vi "AuMT8852B Tester Firmware and Date stamp.vi"(8 "error in (no error)":errorcluster, 11 "VISA session":refnum<visa-resource-name>) -> (0 "error out":errorcluster, 2 "error code":i32, 3 "VISA session out":refnum<visa-resource-name>, 4 "Tester Firmware Date Stamp":T1)   [LabVIEW 2017]
doc: "Anritsu MT8852B Bluetooth Tester\n\nObtains the version and date stamp information for all the modules with the Anritsu Bluetooth test set.\n\nTester Information:\nBase Band boot code date and time stamp.\nBase Band ARM code date and time stamp.\nBase Band FPGA date and time stamp.\nRF FPGA date and time stamp.\nDSP software version number."
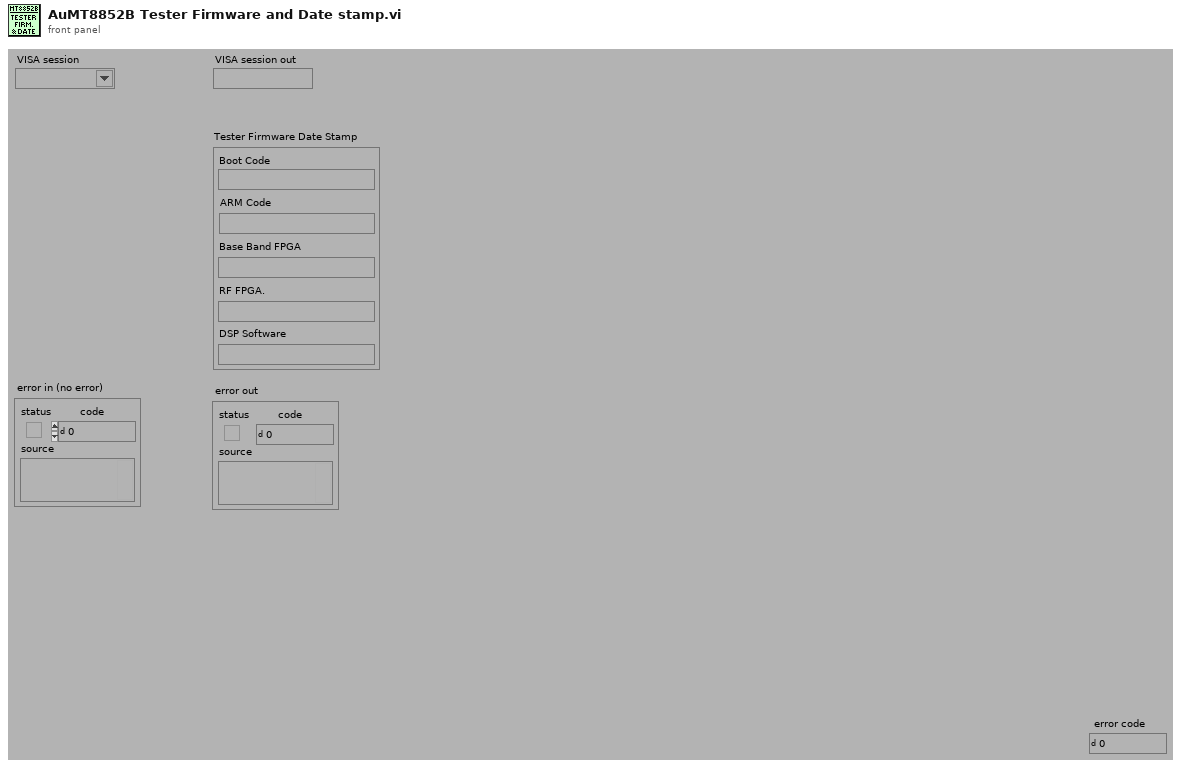
[diagram p1: front panel]
types:
  T1 = cluster{"ARM Code":string, "Base Band FPGA":string, "DSP Software":string, "RF FPGA.":string, "Boot Code":string}
  T2 = enum16{"Simulate", "Range check", "Cache", "Query instrument status"}
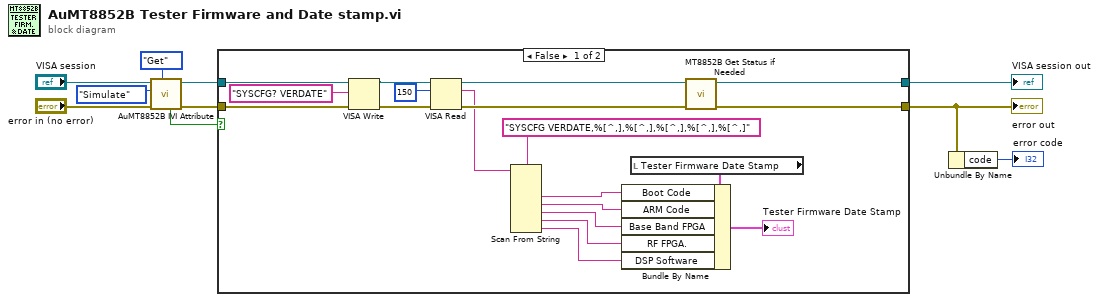
[diagram p0: block diagram]
diagram:
  n1 = call <instrlib>:"AuMT8852B IVI Attribute.vi"("Set/Get (Set)"=enum16{"Set", "Get"}."Get", "error in (no error)"="error in (no error)", "Flag (Simulate)"=T2."Simulate", "VISA session"="VISA session") -> ("error out"=w7:errorcluster, "VISA session out"=w9:refnum<visa-resource-name>, "Value out"=w3:bool)  [unwired: 5 in]
  n2 = case shown="False" w3 {
    tunnel: [w21 w31] -> w10
    tunnel: [w20 w30] -> w1
    tunnel: w9 -> [w28 w31]
    tunnel: w7 -> [w27 w30]
    frame False {
      n3 = VISA Write(VISA resource name=w28, write buffer="SYSCFG? VERDATE" ("write buffer (\"\")"), error in (no error)=w27) -> (VISA resource name out=w26:refnum<visa-resource-name>, error out=w25:errorcluster)  [unwired: 1 out]
      n4 = VISA Read(VISA resource name=w26, byte count=u32 150 ("byte count (0)"), error in (no error)=w25) -> (VISA resource name out=w18:refnum<visa-resource-name>, read buffer=w16:string, error out=w19:errorcluster)  [unwired: 1 out]
      n5 = Scan From String(format string="SYSCFG VERDATE,%[^,],%[^,],%[^,],%[^,],%[^,]" ("write buffer (\"\")"), input string=w16) -> (output 1=w15:string, output 2=w12:string, output 3=w14:string, output 4=w13:string, output 5=w11:string)  [unwired: 7 in, 3 out]
      n6 = local read "Tester Firmware Date Stamp"() -> (w23:T1)
      n7 = Bundle By Name(cluster=w23, "Boot Code"=w15, "ARM Code"=w12, "Base Band FPGA"=w14, "RF FPGA."=w13, "DSP Software"=w11) -> (→"Tester Firmware Date Stamp":T1)
      n8 = call <instrlib>:"MT8852B Get Status if Needed.vi"("error in (no error)"=w19, "VISA session"=w18) -> ("error out"=w20:errorcluster, "VISA session out"=w21:refnum<visa-resource-name>)  [unwired: 8 in]
    }
    frame True {
    }
  }
  "error out" <- w1
  "VISA session out" <- w10
  n9 = Unbundle By Name(w1) -> ("code"=→"error code":i32)
